vi "Serial_Config.vi"() -> (1 "VISA resource name out":refnum<visa-resource-name>, 2 "error out":errorcluster)   [LabVIEW 2018]
uses:
  <vilib>/Instr/_visa.llb/VISA Configure Serial Port (Instr).vi
panel:
  in  "Porta":refnum<visa-resource-name>
  in  "Configurar":bool
  # "Config Serial"
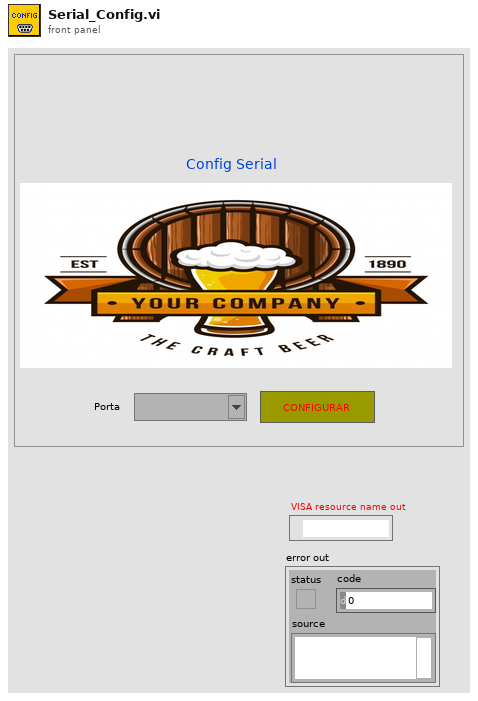
[diagram p1: front panel]
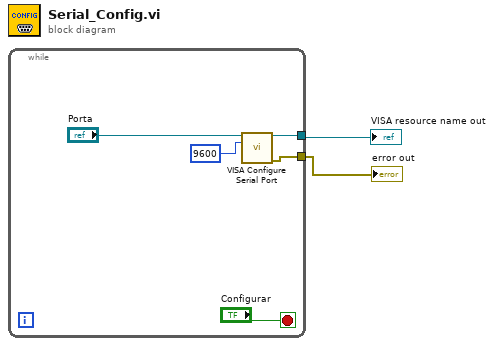
[diagram p0: block diagram]
diagram:
  n1 = while {
    tunnel: [w5] -> w2
    tunnel: [w4] -> w1
    stop <- "Configurar" stop-if-true
    n2 = call-poly "VISA Configure Serial Port"("VISA resource name"="Porta", "baud rate (9600)"=u32 9600) -> ("VISA resource name out"=w5:refnum<visa-resource-name>, "error out"=w4:errorcluster)  [unwired: 12 in]
  }
  "VISA resource name out" <- w2
  "error out" <- w1
